vi "Android_SerialComm.vi"(8 "error in (no error)":errorcluster, 11 "VISA Refnum in":refnum<visa-resource-name>) -> (0 "error out":errorcluster, 2 "Read Buffer":string, 3 "VISA Refnum out":refnum<visa-resource-name>)   [LabVIEW 2015]
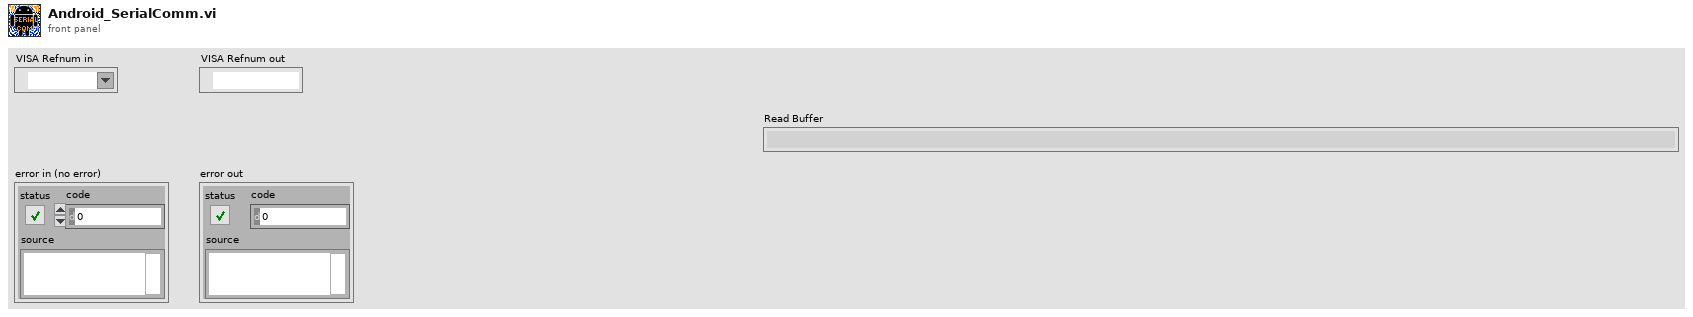
[diagram p1: front panel]
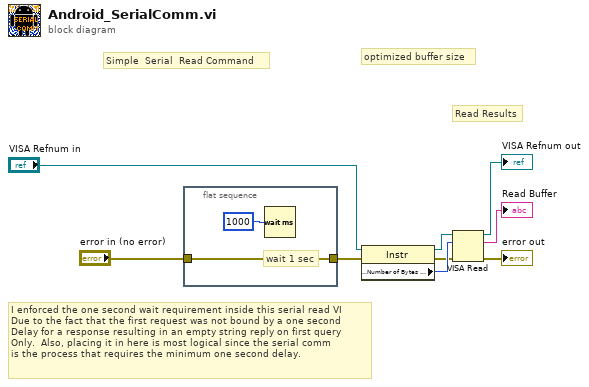
[diagram p0: block diagram]
diagram:
  # "optimized buffer size"
  # "I enforced the one second wait requirement inside this serial read VI \nDue to the fact that the first request was not bound by a one second\nDelay for a response resulting in an empty string reply on first query \nOnly.  Also, placing it in here is most logical since the serial comm\nis the process that requires the minimum one second delay."
  # "Read Results"
  # "Simple  Serial  Read Command"
  n1 = flat-sequence {
    tunnel: "error in (no error)" -> [w10]
    tunnel: [w10] -> w3
    frame #0 {
      # "wait 1 sec"
      n2 = Wait (ms)(milliseconds to wait=u32 1000 ("millisecond multiple")) -> ()  [unwired: 1 out]
    }
  }
  n3 = property class="Instr"(reference="VISA Refnum in", error in=w3) -> (reference out=w6:refnum<visa-resource-name>, error out=w7:errorcluster, "Serial Settings:Number of Bytes at Serial Port"=w8:u32)
  n4 = VISA Read(VISA resource name=w6, byte count=w8, error in (no error)=w7) -> (VISA resource name out=→"VISA Refnum out":refnum<visa-resource-name>, read buffer=→"Read Buffer":string, error out=→"error out":errorcluster)  [unwired: 1 out]
